vi "Custom source-meter - Connect.vi"(8 "Error In":errorcluster, 11 "Source-meter":T2) -> (0 "Error Out":errorcluster, 2 "Result":T4(ring), 3 "Source-meter handle":T1)   [LabVIEW 2019]
doc: "This subVI is meant to perform all operations necessary to establish a connection with your source meter and to initialize it. Your custom settings are made available to you. Remember to return connection status to the Temp handle and Result indicators."
uses:
  Type defs/Source-meter Type Def.ctl
  Custom source-meter settings.ctl
  Type defs/Source-meter handle Type Def.ctl
panel:
  # "Place all operations necessary for connection and initialization of your custom source-meter in this VI"
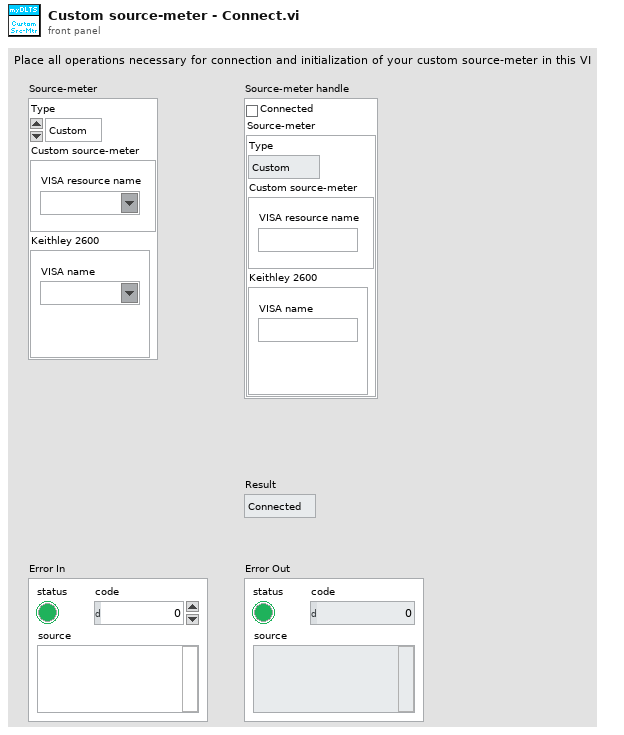
[diagram p1: front panel]
types:
  T1 = typedef "Source-meter handle Type Def.ctl" = cluster{"Connected":bool, "Source-meter":T2}
  T2 = typedef "Source-meter Type Def.ctl" = cluster{"Type":enum16{"Custom", "Keithley 2600"}, "Custom source-meter":T3, "Keithley 2600":cluster{"VISA name":refnum<visa-resource-name>}}
  T3 = typedef "Custom source-meter settings.ctl" = cluster{"VISA resource name":refnum<visa-resource-name>}
  T4 = enum16{"Connected", "Not connected", "Incorrect settings"}
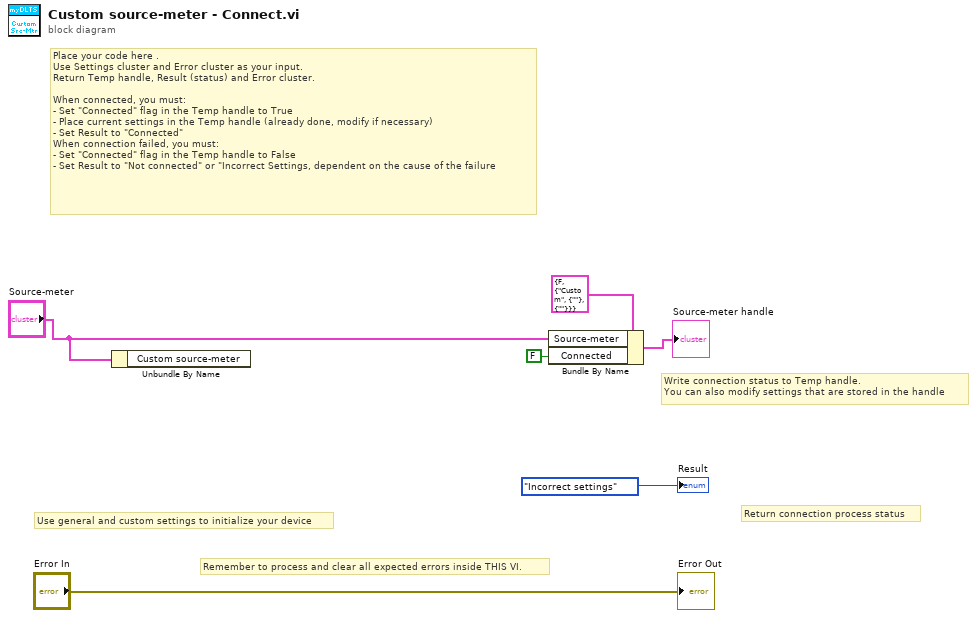
[diagram p0: block diagram]
diagram:
  # "Place your code here .\nUse Settings cluster and Error cluster as your input.\nReturn Temp handle, Result (status) and Error cluster.\n\nWhen connected, you must:\n- Set \"Connected\" flag in the Temp handle to True\n- Place current settings in the Temp handle (already done, modify if necessary)\n- Set Result to \"Connected\"\nWhen connection failed, you must:\n- Set \"Connected\" flag in the Temp handle to False\n- Set Result to \"Not connected\" or \"Incorrect Settings, dependent on the cause of the failure"
  # "Remember to process and clear all expected errors inside THIS VI."
  # "Return connection process status"
  # "Write connection status to Temp handle. \nYou can also modify settings that are stored in the handle"
  # "Use general and custom settings to initialize your device"
  n1 = Unbundle By Name("Source-meter") -> ()  [unwired: 1 out]
  n2 = Bundle By Name(cluster=T1 {"Connected"=FALSE, "Source-meter"={"Type"=enum."Custom", "Custom source-meter"={"VISA resource name"=""}, "Keithley 2600"={"VISA name"=""}}} ("Source-meter handle"), "Source-meter"="Source-meter", "Connected"=FALSE) -> (→"Source-meter handle":T1)
  "Result" <- T4."Incorrect settings" ("Result")
  "Error Out" <- "Error In"
